vi "setJobFilename.vi"(8 "error in (no error)":errorcluster, 10 "Path to Job File":path, 11 "VGS_Job in":refnum<class "VGS_Job.lvclass">) -> (0 "error out":errorcluster, 3 "VGS_Job out":refnum<class "VGS_Job.lvclass">)   [LabVIEW 2022 SP3, in "LV_VGS.lvlib" / "VGS_Job.lvclass"]
uses:
  VGS_Job.lvclass
  VGS_Job.lvclass/VGS_Job.ctl
  C:/Users/Andrey/Documents/GitHub/LV_VGS/vgs_project.dll
  vgs_project.dll
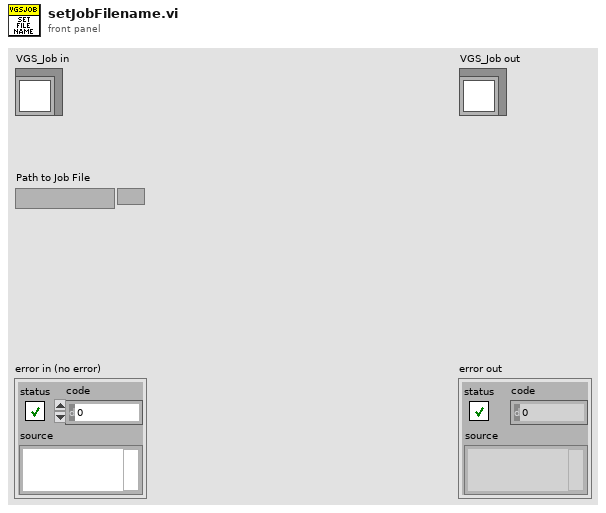
[diagram p1: front panel]
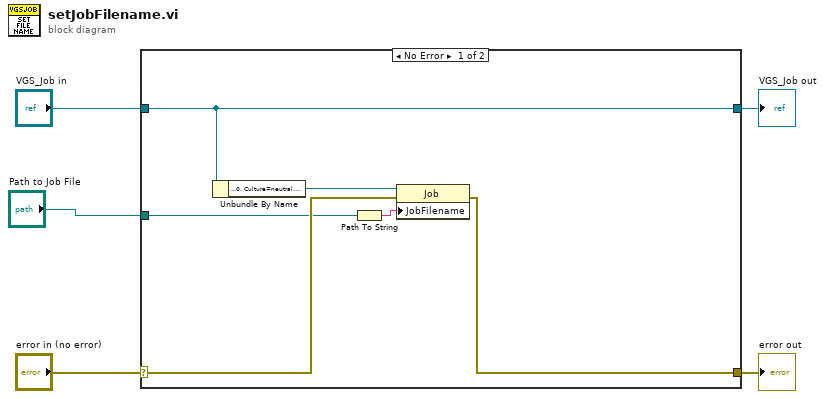
[diagram p0: block diagram]
diagram:
  n1 = case shown="No Error" "error in (no error)" {
    selector: "error in (no error)" -> [w9 w13]
    tunnel: [w8 w13] -> w4
    tunnel: [w11 w12] -> w2
    tunnel: "VGS_Job in" -> [w11 w12]
    tunnel: "Path to Job File" -> [w7 _]
    frame No Error {
      n2 = Unbundle By Name(w11) -> ("Job reference"=w10:refnum<k24>)
      n3 = Path To String(path=w7) -> (string=w6:string)
      n4 = property class="Job"(reference=w10, error in=w9, "JobFilename"=w6) -> (error out=w8:errorcluster)  [unwired: 1 out]
    }
    frame Error {
    }
  }
  "error out" <- w4
  "VGS_Job out" <- w2
